vi "SHAPE_savePaths.vi"(8 "error in (no error)":errorcluster, 9 "SearchType":T1, 10 "Paths":cluster{"Training Data":path}, 11 "BandGlobalOpt in":refnum<class "Shapelets Search GA.lvclass">) -> (0 "error out":errorcluster, 3 "BandGlobalOpt out":refnum<class "Shapelets Search GA.lvclass">)   [LabVIEW 2016, in "Shapelets Search (GA).lvlib" / "Shapelets Search GA.lvclass"]
uses:
  Shapelets Search GA.lvclass
  SHAPE_SearchTypes.ctl
  Shapelets Search GA.lvclass/Shapelets Search GA.ctl
  Shapelets Search (GA).lvlib
panel:
  # "This VI is a part of BCI Design library, http://www.ru-bci.org \nCopyright © 2020, Sotnikov Peter, All rights reserved. License: GNU GPLv3"
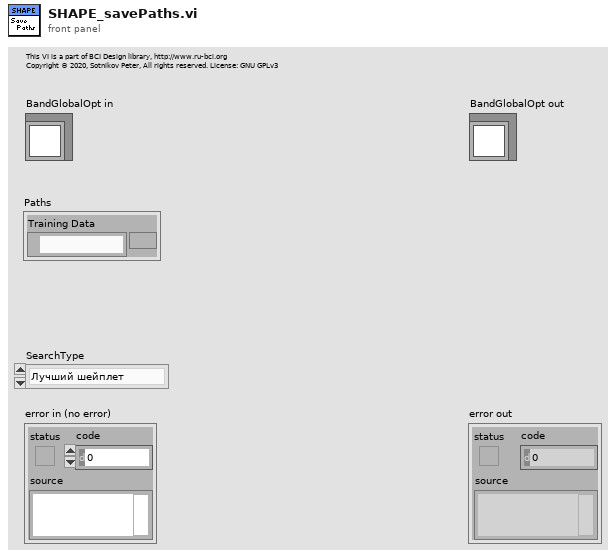
[diagram p1: front panel]
types:
  T1 = typedef "Shapelets Search (GA).lvlib/SHAPE_SearchTypes.ctl" = enum16{"Лучший шейплет", "Набор шейплетов"}
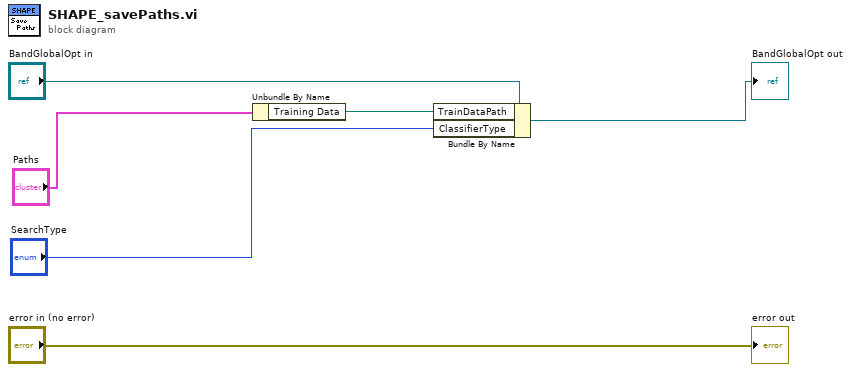
[diagram p0: block diagram]
diagram:
  n1 = Unbundle By Name("Paths") -> ("Training Data"=w2:path)
  n2 = Bundle By Name(cluster="BandGlobalOpt in", "TrainDataPath"=w2, "ClassifierType"="SearchType") -> (→"BandGlobalOpt out":refnum<class "Shapelets Search GA.lvclass">)
  "error out" <- "error in (no error)"
